vi "Do.vi"(8 "error in (no error)":errorcluster, 10 "Actor in":refnum<class "Actor.lvclass">, 11 "Save Test Executive Msg":refnum<class "Save Test Executive Msg.lvclass">) -> (0 "error out":errorcluster, 2 "Actor out":refnum<class "Actor.lvclass">)   [LabVIEW 2017, in "Save Test Executive Msg.lvclass"]
doc: "This VI delivers the message to the actor by calling the appropriate method(s) on the actor."
uses:
  <vilib>/gpm_packages/@cs/Test-executive-builder/Source/Test Executive Builder Model/Test Executive Builder Model Messages/Save Test Executive Msg/Save Test Executive Msg.lvclass
  <vilib>/ActorFramework/Actor/Actor.lvclass
  <vilib>/gpm_packages/@cs/Test-executive-builder/Source/Test Executive Builder Model/Test Executive Builder Model/Test Executive Builder Model.lvclass
  C:/Program Files/National Instruments/LabVIEW 2017/vi.lib/ActorFramework/Actor/Actor.lvclass
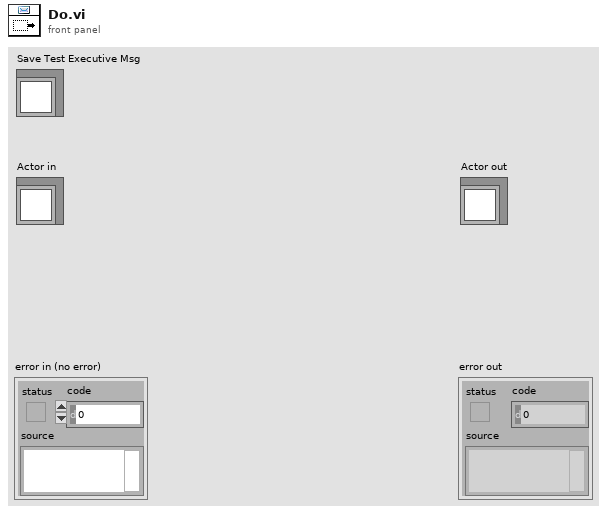
[diagram p1: front panel]
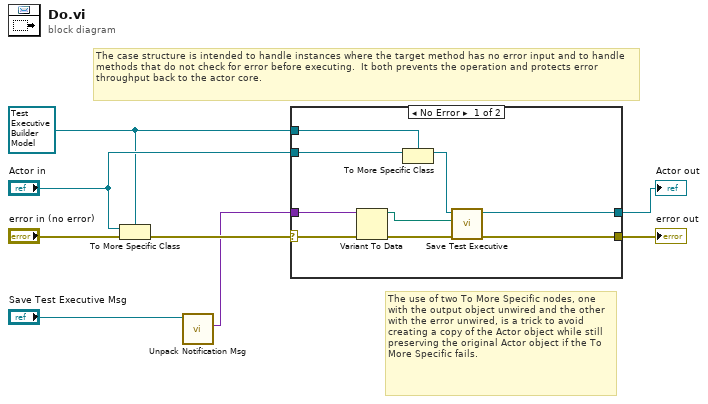
[diagram p0: block diagram]
diagram:
  w3 = refnum<class "Test Executive Builder Model.lvclass"> refnum ("Actor in")
  # "The use of two To More Specific nodes, one with the output object unwired and the other with the error unwired, is a trick to avoid creating a copy of the Actor object while still preserving the original Actor object if the To More Specific fails."
  # "The case structure is intended to handle instances where the target method has no error input and to handle methods that do not check for error before executing.  It both prevents the operation and protects error throughput back to the actor core."
  n1 = To More Specific Class(target class=w3, reference="Actor in", error in="error in (no error)") -> (error out=w7:errorcluster)  [unwired: 1 out]
  n2 = call-dynamic "Unpack Notification Msg.vi"("Notification Msg"="Save Test Executive Msg") -> ("Value"=w1:variant)  [unwired: 8 in, 2 out]
  n3 = case shown="No Error" w7 {
    selector: w7 -> [w12 w19]
    tunnel: [w17 w19] -> w6
    tunnel: [w16 w18] -> w5
    tunnel: "Actor in" -> [w15 w18]
    tunnel: w3 -> [w14 _]
    tunnel: w1 -> [w9 _]
    frame No Error {
      n4 = Variant To Data(error in=w12, Variant=w9) -> (data=w10:path, error out=w11:errorcluster)  [unwired: 1 in]
      n5 = To More Specific Class(target class=w14, reference=w15) -> (specific class reference=w13:refnum<class "Test Executive Builder Model.lvclass">)  [unwired: 1 in, 1 out]
      n6 = call-dynamic "Save Test Executive.vi"("error in (no error)"=w11, "Path"=w10, "Test Executive Builder Model in"=w13) -> ("error out"=w17:errorcluster, "Test Executive Builder Model out"=w16:refnum<class "Test Executive Builder Model.lvclass">)  [unwired: 7 in]
    }
    frame Error {
      # "If type check fails, pass the original object out again."
    }
  }
  "error out" <- w6
  "Actor out" <- w5
